vi "sort filenames.vi"(11 "Image Folder Path":path) -> (3 "Sorted Names":string[](array[string]))   [LabVIEW 2012]
panel:
  out "file number":string
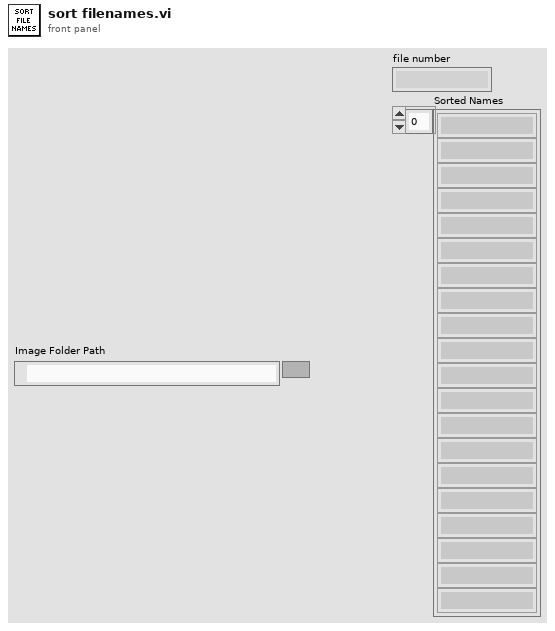
[diagram p1: front panel]
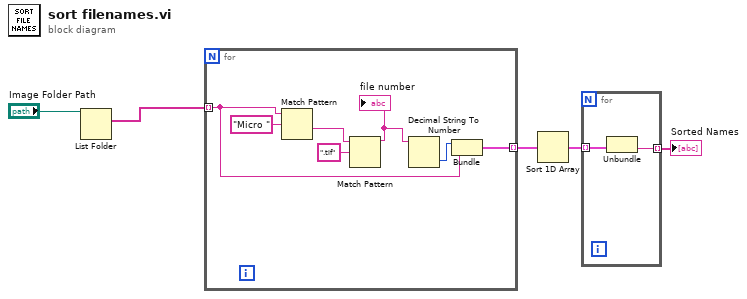
[diagram p0: block diagram]
diagram:
  n1 = List Folder(path="Image Folder Path") -> (filenames=w5:string[])  [unwired: 3 in, 3 out]
  n2 = for {
    tunnel: w5 -> [w7] mode=indexing
    tunnel: [w6] -> w4 mode=indexing
    n3 = Match Pattern(string=w7, regular expression="Micro ") -> (after substring=w10:string)  [unwired: 1 in, 3 out]
    n4 = Match Pattern(string=w10, regular expression=".tif") -> (before substring=w9:string)  [unwired: 1 in, 3 out]
    "file number" <- w9
    n5 = Decimal String To Number(string=w9) -> (number=w8:i32)  [unwired: 2 in, 1 out]
    n6 = Bundle(w8, w7) -> (w6:cluster{i32, string})  [unwired: 1 in]
  }
  n7 = Sort 1D Array(array=w4) -> (sorted array=w3:cluster{i32, string}[])
  n8 = for {
    tunnel: w3 -> [w14] mode=indexing
    tunnel: [w13] -> w2 mode=indexing
    n9 = Unbundle(w14) -> (w13:string)  [unwired: 1 out]
  }
  "Sorted Names" <- w2
